vi "Global - TP Channels.vi"() -> ()   [LabVIEW 2018]
panel:
  in  "TorqueLC":refnum<k21>="ni.var.io://192.168.1.2/EtherCAT/TP/03LC/00RotTrqLC"
  in  "TableLC4":refnum<k21>="ni.var.io://192.168.1.2/EtherCAT/TP/02LC/03TableLC4"
  in  "TableLC3":refnum<k21>="ni.var.io://192.168.1.2/EtherCAT/TP/02LC/02TableLC3"
  in  "TableLC2":refnum<k21>="ni.var.io://192.168.1.2/EtherCAT/TP/02LC/01TableLC2"
  in  "TableLC1":refnum<k21>="ni.var.io://192.168.1.2/EtherCAT/TP/02LC/00TableLC1"
  in  "TablePos":refnum<k21>="ni.var.io://192.168.1.2/EtherCAT/TP/01AI/02TablePos"
  in  "TiltY":refnum<k21>="ni.var.io://192.168.1.2/EtherCAT/TP/01AI/01TiltSensorY"
  in  "TiltX":refnum<k21>="ni.var.io://192.168.1.2/EtherCAT/TP/01AI/00TiltSensorX"
  in  "Encoder0":refnum<k21>="ni.var.io://192.168.1.2/EtherCAT/TP/04DIO/02HEncoder0"
  in  "Encoder2":refnum<k21>="ni.var.io://192.168.1.2/EtherCAT/TP/04DIO/01HEncoder2"
  in  "Encoder1":refnum<k21>="ni.var.io://192.168.1.2/EtherCAT/TP/04DIO/00HEncoder1"
  # "Traveling Plate"
  # "AI"
  # "DIDO"
  # "LC"
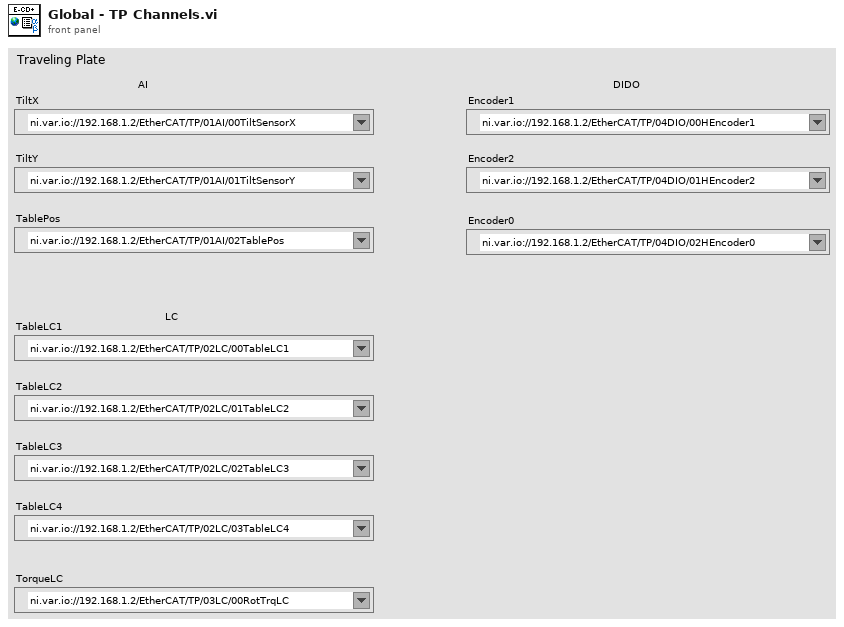
[diagram p1: front panel]
diagram:
